vi "Read In Chain.vi"(11 "Interlock in":refnum<class "Interlock.lvclass">) -> (2 "In Chain":T1, 3 "Interlock out":refnum<class "Interlock.lvclass">)   [LabVIEW 2015, in "Interlocks.lvlib" / "Interlock.lvclass"]
uses:
  Interlock.lvclass
  Controls/Add IL to -Enumerator.ctl
  Interlock.lvclass/Interlock.ctl
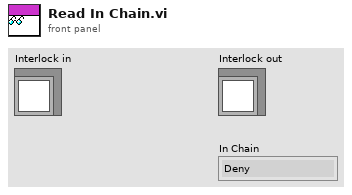
[diagram p1: front panel]
types:
  T1 = typedef "Add IL to -Enumerator.ctl" = enum16{"Deny", "Allow", "None"}
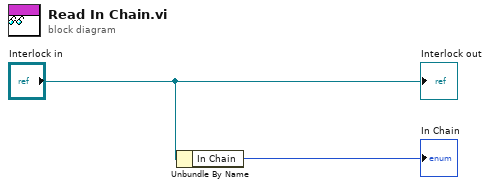
[diagram p0: block diagram]
diagram:
  n1 = Unbundle By Name("Interlock in") -> ("In Chain"=→"In Chain":T1)
  "Interlock out" <- "Interlock in"
